vi "例5-3.vi"() -> ()   [LabVIEW 2019]
uses:
  <vilib>/DAQmx/read.llb/DAQmx Read (Analog 1D Wfm NChan NSamp).vi
  <vilib>/DAQmx/create/channels.llb/DAQmx Create Channel (AI-Voltage-Basic).vi
  <vilib>/DAQmx/configure/timing.llb/DAQmx Timing (Sample Clock).vi
  <vilib>/DAQmx/miscellaneous.llb/DAQmx Fill In Error Info.vi
panel:
  in  "采集通道数":dbl
  in  "物理通道":tag[](array[tag])
  in  "停止":bool
  out "波形图":waveform(dbl)[](graph)
  in  "samples per channel":i32=100 caption="每通道采样"
  in  "rate":dbl=1000.0 caption="速率" format="%0.2f"
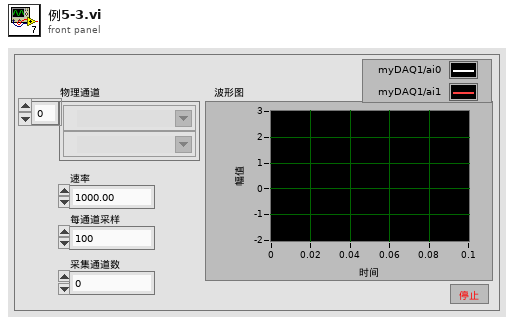
[diagram p1: front panel]
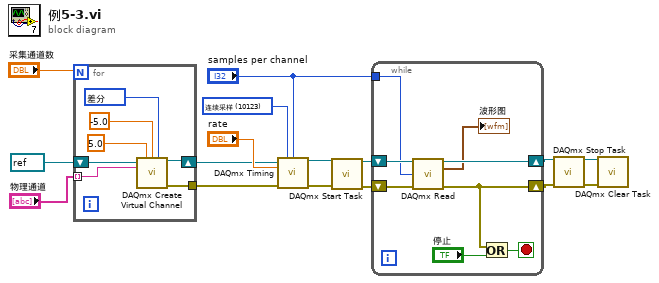
[diagram p0: block diagram]
diagram:
  w15 = 10123 items=["有限采样"=10178, "连续采样"=10123, "硬件定时单点"=12522] ("sample mode")
  n1 = for {
    N: "采集通道数" -> [_]
    tunnel: [w22] -> w13
    shift-right: [w18] -> w3
    shift-left: refnum<k21> refnum ("task in") -> [w19]
    tunnel: "物理通道" -> [w17] mode=indexing
    w23 = 10106 items=["默认"=-1, "RSE"=10083, "NRSE"=10078, "差分"=10106, "伪差分"=12529] ("input terminal configuration")
    n2 = call-poly <vilib>:"DAQmx Create Virtual Channel.vi"("task in"=w19, "maximum value"=5.0, "minimum value"=-5.0, "input terminal configuration"=w23, "physical channels"=w17) -> ("task out"=w18:refnum<k21>, "error out"=w22:errorcluster)  [unwired: 9 in]
  }
  n3 = call-poly <vilib>:"DAQmx Timing.vi"("task/channels in"=w3, "sample mode"=w15, "samples per channel"="samples per channel", "rate"="rate", "error in"=w13) -> ("task out"=w14:refnum<k21>, "error out"=w12:errorcluster)  [unwired: 9 in]
  n4 = call <vilib>:"DAQmx Start Task.vi"("task/channels in"=w14, "error in"=w12) -> ("task out"=w11:refnum<k21>, "error out"=w10:errorcluster)  [unwired: 12 in]
  n5 = while {
    shift-right: [w29] -> w9
    shift-left: w11 -> [w31]
    shift-right: [w26] -> w8
    shift-left: w10 -> [w30]
    tunnel: "samples per channel" -> [w27]
    stop <- w24 stop-if-true
    n6 = call-poly <vilib>:"DAQmx Read.vi"("task/channels in"=w31, "number of samples per channel"=w27, "error in"=w30) -> ("task out"=w29:refnum<k21>, "data"=→"波形图":waveform(dbl)[], "error out"=w26:errorcluster)  [unwired: 10 in]
    n7 = Or(x=w26, y="停止") -> (x .or. y?=w24:bool)
  }
  n8 = call <vilib>:"DAQmx Stop Task.vi"("task/channels in"=w9, "error in"=w8) -> ("task out"=w7:refnum<k21>, "error out"=w6:errorcluster)  [unwired: 12 in]
  n9 = call <vilib>:"DAQmx Clear Task.vi"("task in"=w7, "error in"=w6) -> ()  [unwired: 13 in, 1 out]
